vi "Read payload.vi"(8 "error in (no error)":errorcluster, 11 "JSONWebToken in":refnum<class "JSONWebToken.lvclass">) -> (0 "error out":errorcluster, 2 "payload (JSON)":string, 3 "JSONWebToken out":refnum<class "JSONWebToken.lvclass">)   [LabVIEW 2017, in "JSONWebToken.lvclass"]
uses:
  JSONWebToken.lvclass
  JSONWebToken.lvclass/JSONWebToken.ctl
  <vilib>/JDP Science/JSONtext/JSONtext.lvlib
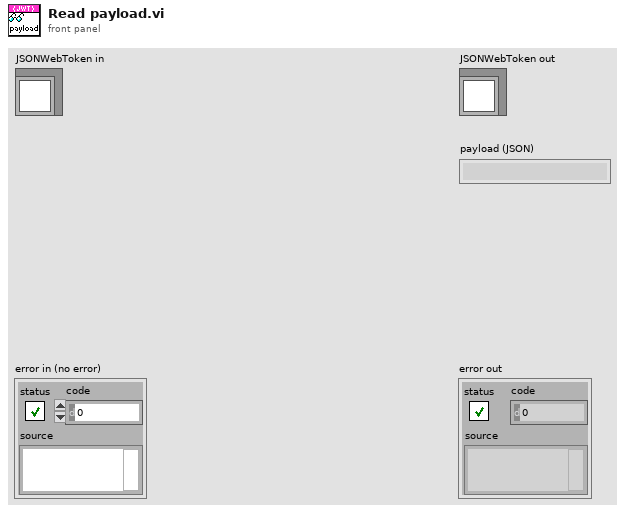
[diagram p1: front panel]
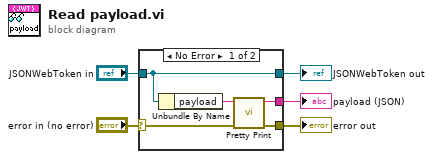
[diagram p0: block diagram]
diagram:
  n1 = case shown="No Error" "error in (no error)" {
    selector: "error in (no error)" -> [w8 w11]
    tunnel: [w7 w11] -> w4
    tunnel: [w10 w12] -> w2
    tunnel: "JSONWebToken in" -> [w10 w12]
    tunnel: [w6 _] -> w1
    frame No Error {
      n2 = Unbundle By Name(w10) -> ("payload"=w9:string)
      n3 = call <vilib>:"Pretty Print.vi"("error in (no error)"=w8, "JSON"=w9) -> ("error out"=w7:errorcluster, "<JSON>"=w6:string)  [unwired: 7 in, 1 out]
    }
    frame Error {
    }
  }
  "error out" <- w4
  "JSONWebToken out" <- w2
  "payload (JSON)" <- w1
